vi "b2g1_sqlite_log_feedflash.vi"(8 "error in (no error)":errorcluster, 10 "nd_vars in":T2, 11 "Output - Cluster b2g1":T1 {"TS-6 [°C]" format="%#.2g"; "TS-5 [°C]" format="%#.2g"; "pHS-1 [pH]" format="%.2g"; "TS-4 [°C]" format="%#.2g"; "FS-2 [l]" format="%.2g"; "FS-1 [l]" format="%.2g"; "DS-1 [bar]" format="%#.2g"; "DFS-1 [l/min]" format="%#.2g"; "FS-3 [l]" format="%.2g"; "DFS-1 [dl]" format="%.0g"}) -> (0 "error out":errorcluster, 3 "nd_vars out":T2)   [LabVIEW 2011]
uses:
  B2G1_nd_vars.ctl
  Output - Cluster b2g1.ctl
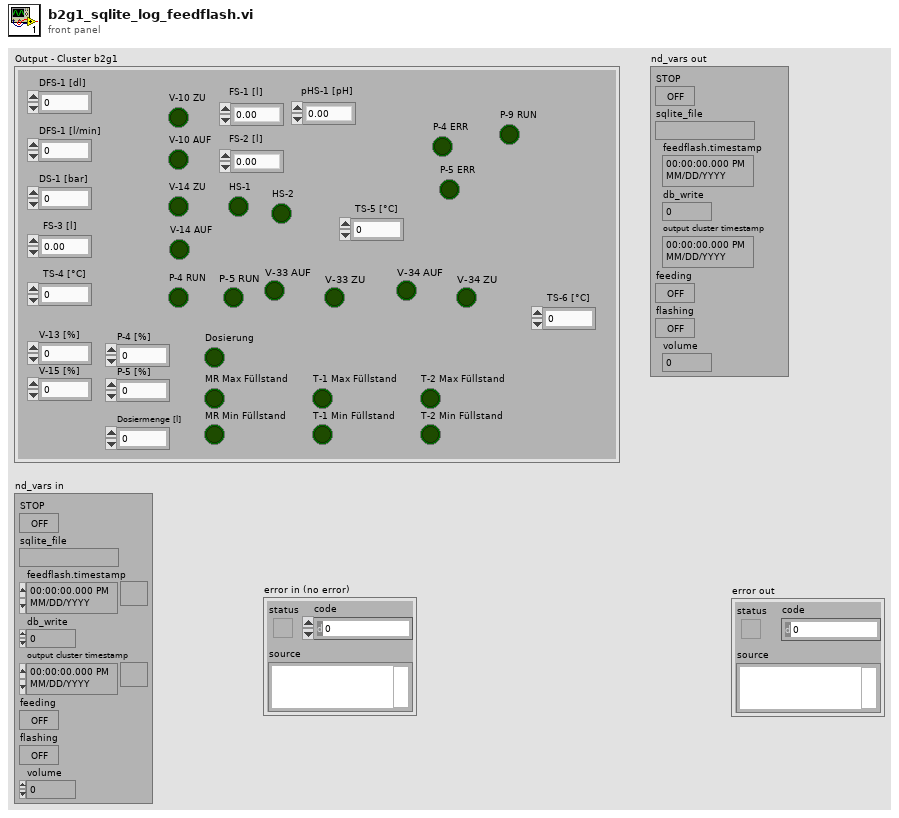
[diagram p1: front panel]
types:
  T1 = typedef "Output - Cluster b2g1.ctl" = cluster{"DFS-1 [dl]":u64, "FS-3 [l]":dbl, "DFS-1 [l/min]":dbl, "DS-1 [bar]":dbl, "V-10 ZU":bool, "V-14 ZU":bool, "FS-1 [l]":dbl, "FS-2 [l]":dbl, "TS-4 [°C]":dbl, "HS-1":bool, "V-13 [%]":u8, "V-15 [%]":u8, "P-4 [%]":u8, "P-5 [%]":u8, "Dosierung":bool, "MR Max Füllstand":bool, "MR Min Füllstand":bool, "Dosiermenge [l]":sgl, "V-14 AUF":bool, "V-10 AUF":bool, "T-1 Max Füllstand":bool, "T-1 Min Füllstand":bool, "T-2 Max Füllstand":bool, "T-2 Min Füllstand":bool, "pHS-1 [pH]":dbl, "P-4 RUN":bool, "P-5 RUN ":bool, "V-33 AUF":bool, "V-33 ZU":bool, "V-34 AUF":bool, "V-34 ZU":bool, "P-4 ERR":bool, "P-5 ERR":bool, "TS-5 [°C]":dbl, "TS-6 [°C]":dbl, "P-9 RUN":bool, "HS-2":bool}
  T2 = typedef "B2G1_nd_vars.ctl" = cluster{"STOP":bool, "sqlite_file":string, "feedflash.timestamp":timestamp, "db_write":i64, "output cluster timestamp":timestamp, "feeding":bool, "flashing":bool, "volume":u64}
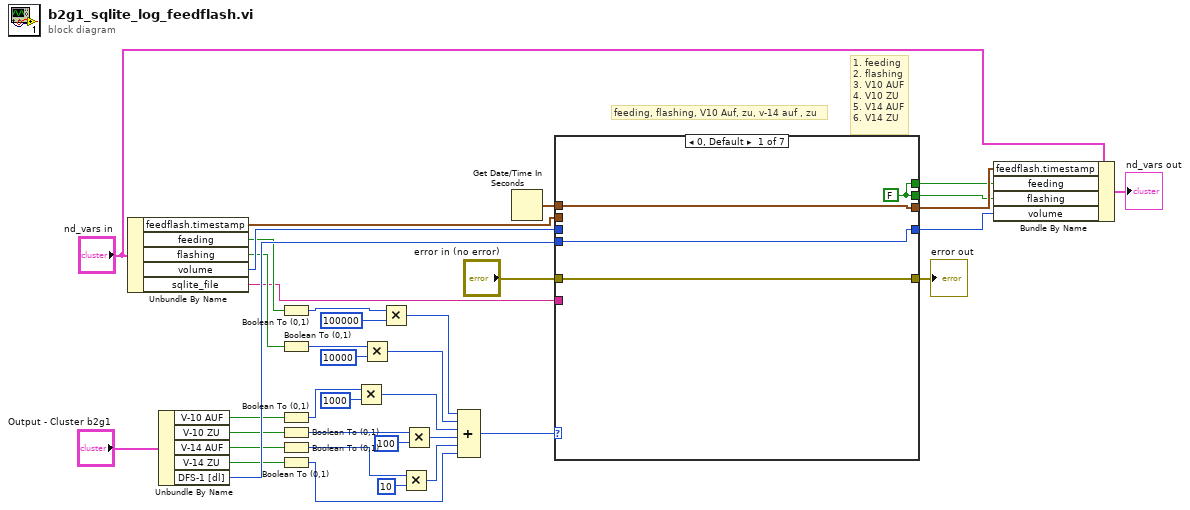
[diagram p0: block diagram]
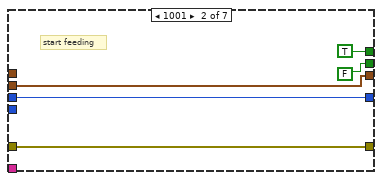
[diagram p2: hidden frame]
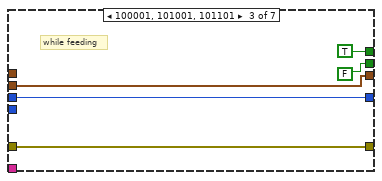
[diagram p3: hidden frame]
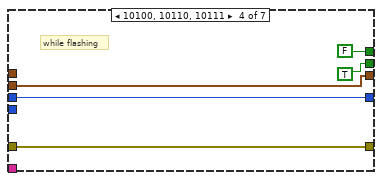
[diagram p4: hidden frame]
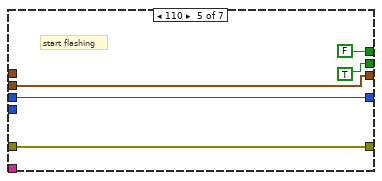
[diagram p5: hidden frame]
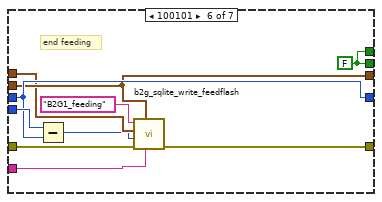
[diagram p6: hidden frame]
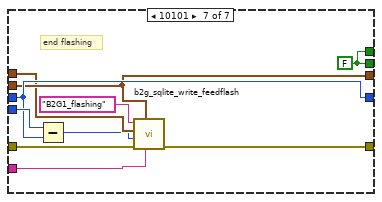
[diagram p7: hidden frame]
diagram:
  # "1. feeding\n2. flashing\n3. V10 AUF\n4. V10 ZU\n5. V14 AUF\n6. V14 ZU"
  # "feeding, flashing, V10 Auf, zu, v-14 auf , zu"
  n1 = Unbundle By Name("nd_vars in") -> ("feedflash.timestamp"=w35:timestamp, "feeding"=w11:bool, "flashing"=w12:bool, "volume"=w34:u64, "sqlite_file"=w1:string)
  n2 = Unbundle By Name("Output - Cluster b2g1") -> ("V-10 AUF"=w7:bool, "V-10 ZU"=w8:bool, "V-14 AUF"=w9:bool, "V-14 ZU"=w10:bool, "DFS-1 [dl]"=w33:u64)
  n3 = Boolean To (0,1)(Boolean=w11) -> (0, 1=w14:i16)
  n4 = Boolean To (0,1)(Boolean=w12) -> (0, 1=w13:i16)
  n5 = Boolean To (0,1)(Boolean=w7) -> (0, 1=w17:i16)
  n6 = Boolean To (0,1)(Boolean=w8) -> (0, 1=w18:i16)
  n7 = Boolean To (0,1)(Boolean=w9) -> (0, 1=w19:i16)
  n8 = Boolean To (0,1)(Boolean=w10) -> (0, 1=w23:i16)
  n9 = Multiply(x=w17, y=1000) -> (x*y=w20:i32)
  n10 = Multiply(x=w13, y=10000) -> (x*y=w16:i32)
  n11 = Multiply(x=w14, y=100000) -> (x*y=w15:i32)
  n12 = Multiply(x=w19, y=10) -> (x*y=w22:i32)
  n13 = Multiply(x=w18, y=100) -> (x*y=w21:i32)
  n14 = Compound Arithmetic op=ADD(w15, w16, w20, w21, w22, w23) -> (w29:i32)
  n15 = Get Date/Time In Seconds() -> (seconds since 1Jan1904=w37:timestamp)
  n16 = case shown="0, Default" w29 {
    tunnel: [w41 TRUE TRUE FALSE FALSE w62 w72] -> w30
    tunnel: [w41 FALSE FALSE TRUE TRUE w62 w72] -> w31
    tunnel: [w40 w45 w50 w55 w60 w70 w80] -> w32
    tunnel: w33 -> [w40 _ _ _ _ w71 w81]
    tunnel: w34 -> [_ w45 w50 w55 w60 w70 w80]
    tunnel: w35 -> [_ w43 w48 w53 w58 w69 w79]
    tunnel: [w39 w43 w48 w53 w58 w69 w79] -> w36
    tunnel: w37 -> [w39 _ _ _ _ w68 w78]
    tunnel: "error in (no error)" -> [w38 w42 w47 w52 w57 w65 w75]
    tunnel: [w38 w42 w47 w52 w57 w64 w74] -> w2
    tunnel: w1 -> [_ _ _ _ _ w63 w73]
    frame 0, Default {
      w41 = FALSE
    }
    frame 1001 {
      # "start feeding"
    }
    frame 100001, 101001, 101101 {
      # "while feeding"
    }
    frame 10100, 10110, 10111 {
      # "while flashing"
    }
    frame 110 {
      # "start flashing"
    }
    frame 100101 {
      w62 = FALSE
      # "end feeding"
      n17 = Subtract(x=w71, y=w70) -> (x-y=w67:u64)
      n18 = call "b2g_sqlite_write_feedflash.vi"("Database File"=w63, "feedflash.timestamp"=w69, "error in (no error)"=w65, "Numeric"=w67, "seconds since 1Jan1904"=w68, "SQL Query"="B2G1_feeding") -> ("error out"=w64:errorcluster)  [unwired: 5 in]
    }
    frame 10101 {
      w72 = FALSE
      # "end flashing"
      n19 = Subtract(x=w81, y=w80) -> (x-y=w77:u64)
      n20 = call "b2g_sqlite_write_feedflash.vi"("Database File"=w73, "feedflash.timestamp"=w79, "error in (no error)"=w75, "Numeric"=w77, "seconds since 1Jan1904"=w78, "SQL Query"="B2G1_flashing") -> ("error out"=w74:errorcluster)  [unwired: 5 in]
    }
  }
  "error out" <- w2
  n21 = Bundle By Name(cluster="nd_vars in", "feedflash.timestamp"=w36, "feeding"=w30, "flashing"=w31, "volume"=w32) -> (→"nd_vars out":T2)
